vi "9_ВПМассивыДанных.vi"() -> ()   [LabVIEW 2016]
panel:
  out "Массив попарно умноженных чисел":dbl[](array[numeric])
  in  "Входной массив":dbl[](array[numeric])
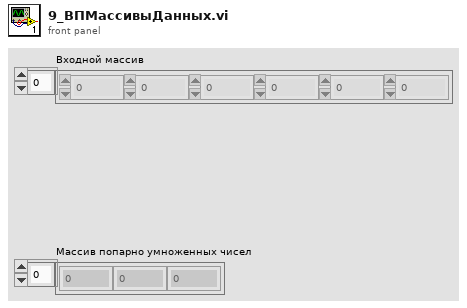
[diagram p1: front panel]
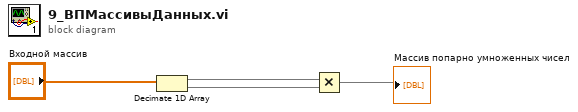
[diagram p0: block diagram]
diagram:
  n1 = Decimate 1D Array("Входной массив") -> (w3:dbl[], w2:dbl[])
  n2 = Multiply(x=w3, y=w2) -> (x*y=→"Массив попарно умноженных чисел":dbl[])
